vi "MF-101 Analog Input.vi"() -> ()   [LabVIEW 8.6]
uses:
  <libdir>/resource/objmgr/ueidaq.rc
  vi.lib/UeiDaq/UeiDaqCreateAISession.vi
  vi.lib/UeiDaq/UeiDaqConfigureTimingForSimpleIO.vi
  vi.lib/UeiDaq/UeiDaqReadOneScaledScan.vi
panel:
  out "Serial Number":string
  out "Name":string
  out "Voltage Divider":i32[](array[ring]) items=["Disable", "Enable"]
  out "Min Range":dbl[](array[numeric])
  out "Max Range":dbl[](array[numeric])
  in  "max range (V)":T1(ring)
  in  "min range (V)":T2(ring)
  out "gain":dbl[](array[numeric])
  in  "data pts":u32
  in  "Analog Input Mode":enum16{"Differential", "Single-Ended"}(ring)
  in  "timeout (ms)":u32
  in  "AI Resource":string
  out "scans":u32
  out "Waveform Chart":dbl[][](graph)
  in  "Refresh rate (ms)":u32
  in  "stop":bool
  # "MF-101 Analog Input Test"
  # "ranges:\n\n     Low  V              High V    \n0.15625 (G64)        1.25 (G64)\n0.625 (G16)             5 (G16)\n   2.5 (G4)              20 (G4)\n    10 (G1)               80 (G1)"
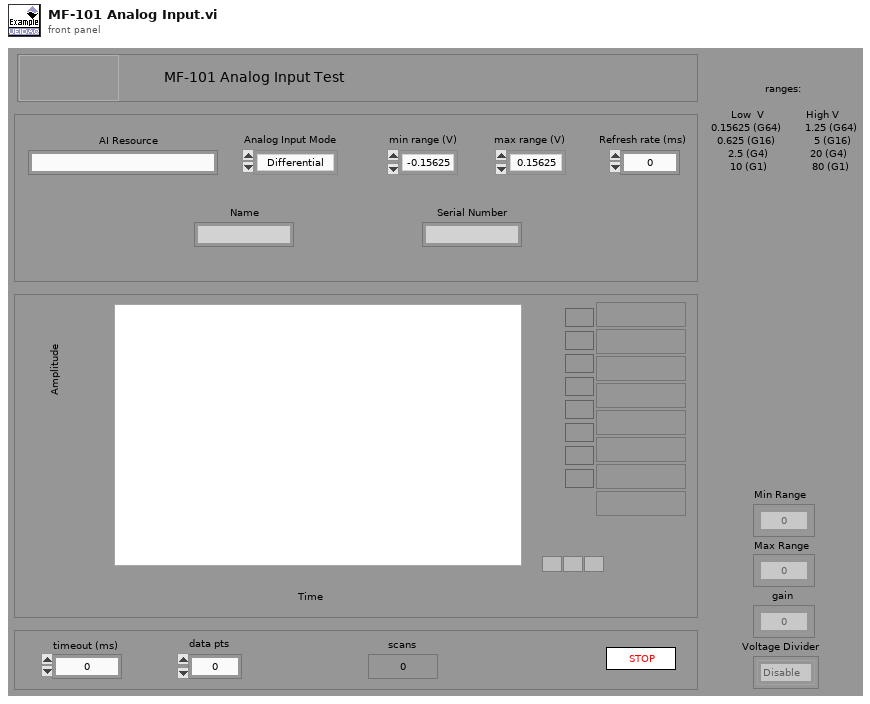
[diagram p1: front panel]
types:
  T1 = enum16{"0.15625", "0.625", "1.25", "2.5", "5", "10", "20", "80"}
  T2 = enum16{"-0.15625", "-0.625", "-1.25", "-2.5", "-5", "-10", "-20", "-80"}
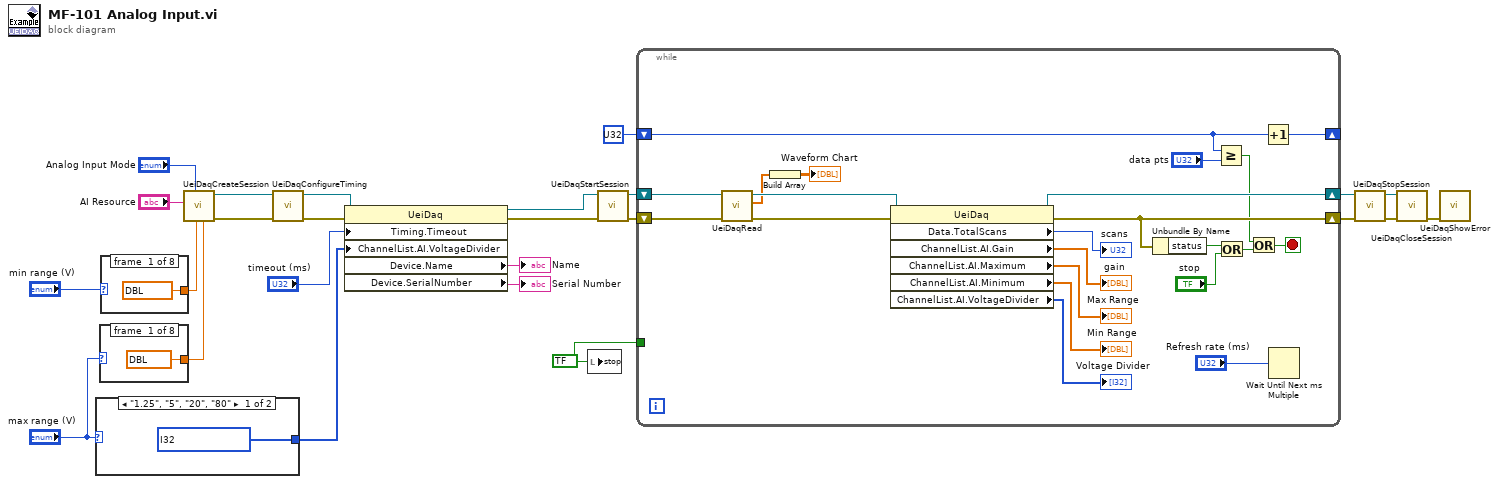
[diagram p0: block diagram]
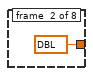
[diagram p2: hidden frame]
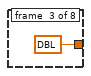
[diagram p3: hidden frame]
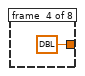
[diagram p4: hidden frame]
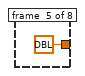
[diagram p5: hidden frame]
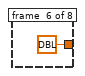
[diagram p6: hidden frame]
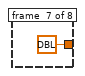
[diagram p7: hidden frame]
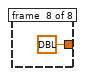
[diagram p8: hidden frame]
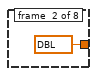
[diagram p9: hidden frame]
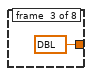
[diagram p10: hidden frame]
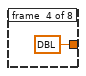
[diagram p11: hidden frame]
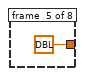
[diagram p12: hidden frame]
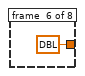
[diagram p13: hidden frame]
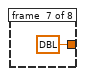
[diagram p14: hidden frame]
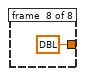
[diagram p15: hidden frame]
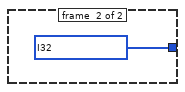
[diagram p16: hidden frame]
diagram:
  w3 = bool ? ("stop")
  n1 = case shown="\"1.25\", \"5\", \"20\", \"80\"" "max range (V)" {
    tunnel: [w26 w27] -> w16
    frame #0 {
      w26 = i32[] ? items=["Disable", "Enable"] ("Channel List:Analog Input:Voltage Divider")
    }
    frame #1 {
      w27 = i32[] ? items=["Disable", "Enable"] ("Channel List:Analog Input:Voltage Divider")
    }
  }
  n2 = case shown="\"10\"" "max range (V)" {
    tunnel: [dbl ? dbl ? dbl ? dbl ? dbl ? dbl ? dbl ? dbl ?] -> w12
    frame #0 {
    }
    frame #1 {
    }
    frame #2 {
    }
    frame #3 {
    }
    frame #4 {
    }
    frame #5 {
    }
    frame #6 {
    }
    frame #7 {
    }
  }
  n3 = case shown="\"-10\"" "min range (V)" {
    tunnel: [dbl ? dbl ? dbl ? dbl ? dbl ? dbl ? dbl ? dbl ?] -> w14
    frame #0 {
    }
    frame #1 {
    }
    frame #2 {
    }
    frame #3 {
    }
    frame #4 {
    }
    frame #5 {
    }
    frame #6 {
    }
    frame #7 {
    }
  }
  n4 = call-poly "UeiDaqCreateSession.vi"("Maximum range"=w12, "Minimum range"=w14, "Analog Input Mode"="Analog Input Mode", "Resource"="AI Resource") -> ("error out"=w23:errorcluster, "UeiDaq Refnum Out"=w24:refnum<k20>)  [unwired: 6 in]
  n5 = call-poly "UeiDaqConfigureTiming.vi"("error in (no error)"=w23, "UeiDaq Refnum In"=w24) -> ("error out"=w21:errorcluster, "UeiDaq Refnum Out"=w20:refnum<k20>)  [unwired: 1 in, 7 out]
  n6 = property class="UeiDaq"(reference=w20, error in=w21, "Timing.Timeout"="timeout (ms)", "ChannelList.AI.VoltageDivider"=w16) -> (reference out=w10:refnum<k20>, error out=w11:errorcluster, "Device.Name"=→"Name":string, "Device.SerialNumber"=→"Serial Number":string)
  n7 = local write "stop"(w3) -> ()
  n8 = call "UeiDaqStartSession.vi"("error in (no error)"=w11, "UeiDaq Refnum In"=w10) -> ("error out"=w8:errorcluster, "UeiDaq Refnum Out"=w9:refnum<k20>)  [unwired: 8 in]
  n9 = while {
    shift-right: [w64] -> w5
    shift-left: w8 -> [w48]
    shift-right: [w65] -> w7
    shift-left: w9 -> [w49]
    shift-right: [w56] -> _
    shift-left: u32 ? -> [w50]
    tunnel: w3 -> [_]
    stop <- w59 stop-if-true
    n10 = call-poly "UeiDaqRead.vi"("error in (no error)"=w48, "UeiDaq Refnum In"=w49) -> ("error out"=w47:errorcluster, "Scaled Data"=w44:dbl[], "UeiDaq Refnum Out"=w46:refnum<k20>)  [unwired: 7 out]
    n11 = Build Array(w44) -> (→"Waveform Chart":dbl[][])
    n12 = property class="UeiDaq"(reference=w46, error in=w47) -> (reference out=w65:refnum<k20>, error out=w64:errorcluster, "Data.TotalScans"=→"scans":u32, "ChannelList.AI.Gain"=→"gain":dbl[], "ChannelList.AI.Maximum"=→"Max Range":dbl[], "ChannelList.AI.Minimum"=→"Min Range":dbl[], "ChannelList.AI.VoltageDivider"=→"Voltage Divider":i32[])
    n13 = Unbundle By Name(w64) -> ("status"=w63:bool)
    n14 = Greater Or Equal?(x=w50, y="data pts") -> (x >= y?=w57:bool)
    n15 = Or(x=w63, y="stop") -> (x .or. y?=w58:bool)
    n16 = Or(x=w57, y=w58) -> (x .or. y?=w59:bool)
    n17 = Increment(x=w50) -> (x+1=w56:u32)
    n18 = Wait Until Next ms Multiple(millisecond multiple="Refresh rate (ms)") -> ()  [unwired: 1 out]
  }
  n19 = call "UeiDaqStopSession.vi"("error in (no error)"=w5, "UeiDaq Refnum In"=w7) -> ("error out"=w4:errorcluster, "UeiDaq Refnum Out"=w6:refnum<k20>)  [unwired: 8 in]
  n20 = call "UeiDaqCloseSession.vi"("error in (no error)"=w4, "UeiDaq Refnum In"=w6) -> ("error out"=w25:errorcluster)  [unwired: 1 in, 8 out]
  n21 = call "UeiDaqShowError.vi"("error in (no error)"=w25) -> ()  [unwired: 2 in, 9 out]
